vi "Create Build Info.vi"(6 "Project Path (Autodetect)":path, 8 "error in (no error)":errorcluster, 9 "Build Spec":string, 10 "Target":string, 11 "Builder in":refnum<class "Builder.lvclass">) -> (0 "error out":errorcluster, 2 "Build Info":T1, 3 "Builder out":refnum<class "Builder.lvclass">)   [LabVIEW 2020, in "Builder Tools.lvlib" / "Builder.lvclass"]
uses:
  Builder.lvclass
  Builder.lvclass/Builder.ctl
  Build Info.ctl
  Builder Tools.lvlib
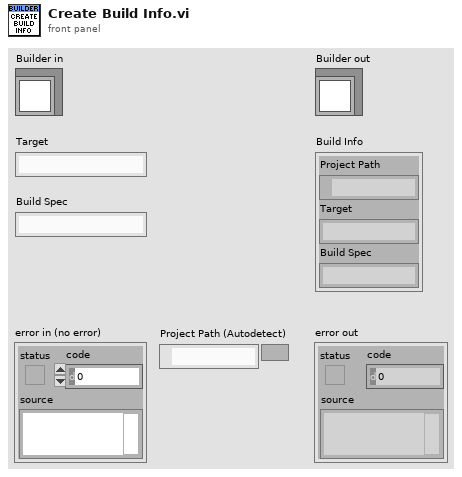
[diagram p1: front panel]
types:
  T1 = typedef "Builder Tools.lvlib/Build Info.ctl" = cluster{"Project Path":path, "Target":string, "Build Spec":string}
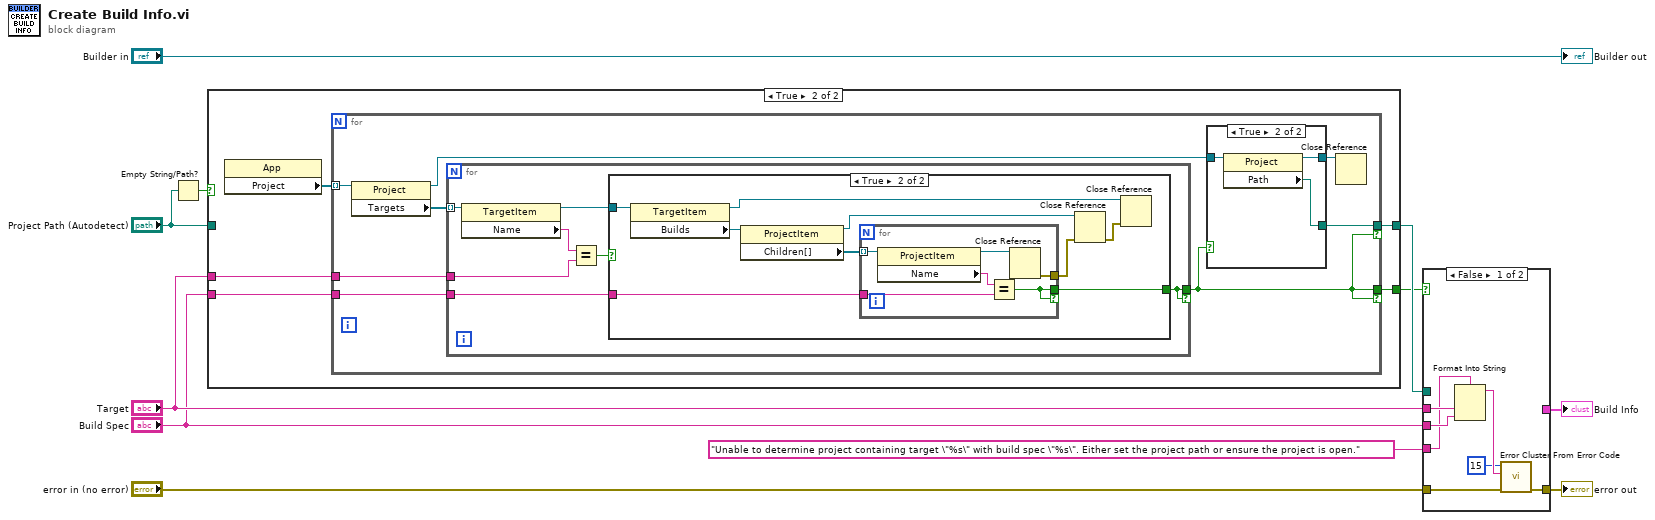
[diagram p0: block diagram]
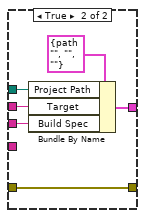
[diagram p2: hidden frame]
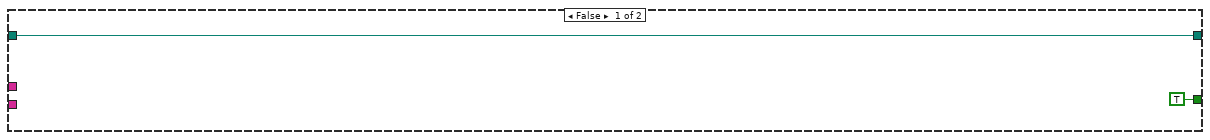
[diagram p3: hidden frame]
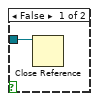
[diagram p5: hidden frame]
diagram:
  n1 = Empty String/Path?(string/path="Project Path (Autodetect)") -> (empty?=w10:bool)
  n2 = case shown="True" w10 {
    tunnel: "Project Path (Autodetect)" -> [w13 _]
    tunnel: "Target" -> [_ w17]
    tunnel: "Build Spec" -> [_ w16]
    tunnel: [w13 w15] -> w5
    tunnel: [TRUE w14] -> w4
    frame False {
    }
    frame True {
      n3 = property class="App"() -> ("Project"=w18:refnum<vi>[])  [unwired: 2 in, 2 out]
      n4 = for {
        tunnel: w18 -> [w26] mode=indexing
        tunnel: w17 -> [w24]
        tunnel: w16 -> [w23]
        tunnel: [w20] -> w14 if=w20
        tunnel: [w21] -> w15 if=w20
        n5 = property class="Project"(reference=w26) -> (reference out=w22:refnum<vi>, "Targets"=w25:refnum<vi>[])  [unwired: 1 in, 1 out]
        n6 = for {
          tunnel: w25 -> [w37] mode=indexing
          tunnel: w24 -> [w35]
          tunnel: w23 -> [w32]
          tunnel: [w31] -> w20 if=w31
          n7 = property class="TargetItem"(reference=w37) -> (reference out=w33:refnum<vi>, "Name"=w36:string)  [unwired: 1 in, 1 out]
          n8 = Equal?(x=w36, y=w35) -> (x = y?=w34:bool)
          n9 = case shown="True" w34 {
            tunnel: w33 -> [w38 w47]
            tunnel: w32 -> [_ w44]
            tunnel: [_ w39] -> w31
            frame False {
              n10 = Close Reference(reference=w38) -> ()  [unwired: 1 in, 1 out]
            }
            frame True {
              n11 = property class="TargetItem"(reference=w47) -> (reference out=w40:refnum<vi>, "Builds"=w46:refnum<vi>)  [unwired: 1 in, 1 out]
              n12 = property class="ProjectItem"(reference=w46) -> (reference out=w42:refnum<vi>, "Children[]"=w45:refnum<vi>[])  [unwired: 1 in, 1 out]
              n13 = for {
                tunnel: w45 -> [w53] mode=indexing
                tunnel: w44 -> [w52]
                tunnel: [w50] -> w39 if=w50
                tunnel: [w48] -> w43
                n14 = property class="ProjectItem"(reference=w53) -> (reference out=w49:refnum<vi>, "Name"=w51:string)  [unwired: 1 in, 1 out]
                n15 = Equal?(x=w51, y=w52) -> (x = y?=w50:bool)
                n16 = Close Reference(reference=w49) -> (error out=w48:errorcluster)  [unwired: 1 in]
              }
              n17 = Close Reference(reference=w42, error in (no error)=w43) -> (error out=w41:errorcluster)
              n18 = Close Reference(reference=w40, error in (no error)=w41) -> ()  [unwired: 1 out]
            }
          }
        }
        n19 = case shown="True" w20 {
          tunnel: w22 -> [w27 w30]
          tunnel: [_ w29] -> w21
          tunnel: [w27 w28] -> w19
          frame False {
          }
          frame True {
            n20 = property class="Project"(reference=w30) -> (reference out=w28:refnum<vi>, "Path"=w29:path)  [unwired: 1 in, 1 out]
          }
        }
        n21 = Close Reference(reference=w19) -> ()  [unwired: 1 in, 1 out]
      }
    }
  }
  n22 = case shown="False" w4 {
    tunnel: [_ w65] -> w8
    tunnel: "Target" -> [w60 w64]
    tunnel: "Build Spec" -> [w59 w63]
    tunnel: w5 -> [_ w62]
    tunnel: "Unable to determine project containing target \"%s\" with build spec \"%s\". Either set the project path or ensure the project is open." -> [w58 _]
    tunnel: [w55 w61] -> w2
    tunnel: "error in (no error)" -> [w54 w61]
    frame False {
      n23 = Format Into String(format string=w58, w60, w59) -> (resulting string=w57:string)  [unwired: 2 in, 1 out]
      n24 = call <vilib>:"Error Cluster From Error Code.vi"("error in (no error)"=w54, "error message (\"\")"=w57, "error code (0)"=15) -> ("error out"=w55:errorcluster)  [unwired: 6 in]
    }
    frame True {
      n25 = Bundle By Name(cluster=T1 {"Project Path"=path "", "Target"="", "Build Spec"=""} ("Build Info"), "Project Path"=w62, "Target"=w64, "Build Spec"=w63) -> (w65:T1)
    }
  }
  "error out" <- w2
  "Build Info" <- w8
  "Builder out" <- "Builder in"
